vi "KE6221 -- Get Output Response.vi"(0 "6221 Resource In":refnum<visa-resource-name>, 1 "Check For SCPI Errors? (T)":bool=TRUE, 11 "error in (no error)":errorcluster) -> (4 "6221 Resource Out (dupl)":refnum<visa-resource-name>, 8 "KE6221 Output Response":T1=enum."Slow", 15 "error out":errorcluster)   [LabVIEW 2019, in "Keithley 622x.lvlib"]
doc: "Returns the output response speed for the 6221. If 'Fast' is returned, the output bandwidth increases to 1MHz. If 'Slow' is returned, the 6221 behaves the same as the 6220."
uses:
  Keithley 622x.lvlib
  Typedefs/KE6221 -- Output Response.ctl
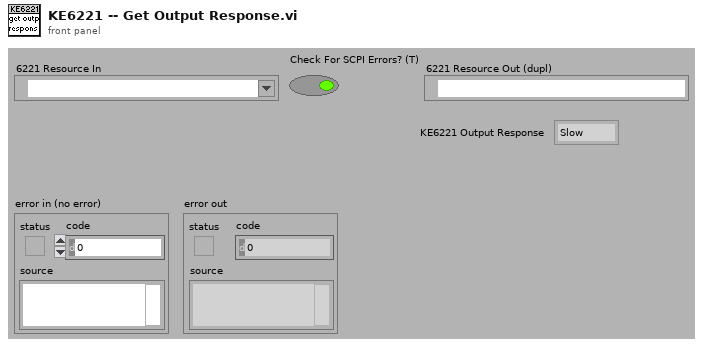
[diagram p1: front panel]
types:
  T1 = typedef "Keithley 622x.lvlib/KE6221 -- Output Response.ctl" = enum16{"Fast", "Slow"}
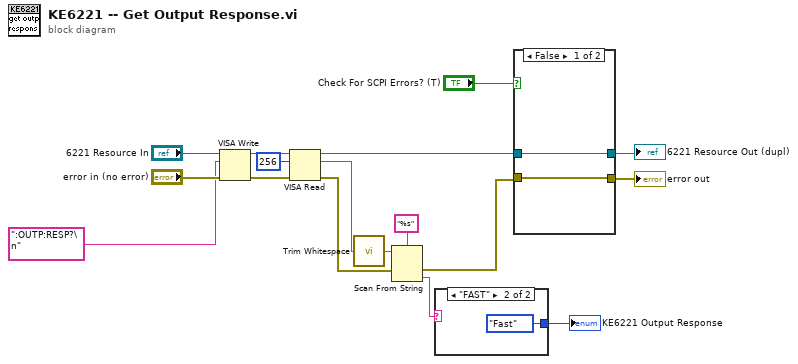
[diagram p0: block diagram]
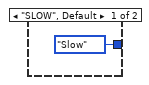
[diagram p2: hidden frame]
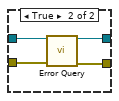
[diagram p3: hidden frame]
diagram:
  n1 = VISA Write(VISA resource name="6221 Resource In", write buffer=":OUTP:RESP?\n" ("format string"), error in (no error)="error in (no error)") -> (VISA resource name out=w11:refnum<visa-resource-name>, error out=w10:errorcluster)  [unwired: 1 out]
  n2 = VISA Read(VISA resource name=w11, byte count=u32 256, error in (no error)=w10) -> (VISA resource name out=w4:refnum<visa-resource-name>, read buffer=w6:string, error out=w8:errorcluster)  [unwired: 1 out]
  n3 = call <vilib>:"Trim Whitespace.vi"("string"=w6) -> ("trimmed string"=w3:string)  [unwired: 1 in]
  n4 = Scan From String(format string="%s", input string=w3, error in=w8) -> (error out=w5:errorcluster, output 1=w2:string)  [unwired: 2 in, 2 out]
  n5 = case shown="\"FAST\"" w2 {
    tunnel: [KE6221_--_Output_Response."Slow" ("KE6221 Output Response") KE6221_--_Output_Response."Fast" ("KE6221 Output Response")] -> w1
    frame "SLOW", Default {
    }
    frame "FAST" {
    }
  }
  "KE6221 Output Response" <- w1
  n6 = case shown="False" "Check For SCPI Errors? (T)" {
    tunnel: w4 -> [w21 w25]
    tunnel: w5 -> [w20 w24]
    tunnel: [w20 w23] -> w13
    tunnel: [w21 w22] -> w14
    frame False {
    }
    frame True {
      n7 = call "Error Query.vi"("VISA Resource In"=w25, "error in (no error)"=w24) -> ("VISA Resource Out (dupl)"=w22:refnum<visa-resource-name>, "error out"=w23:errorcluster)  [unwired: 10 in, 2 out]
    }
  }
  "6221 Resource Out (dupl)" <- w14
  "error out" <- w13
